vi "Write configuration.vi"(8 "error in (no error)":errorcluster, 10 "configuration":refnum<class "CEF_serializable configuration.lvclass">, 11 "DIO Instrument":refnum<class "Digital IO Instrument.lvclass">) -> (0 "error out":errorcluster, 3 "DIO Instrument out":refnum<class "Digital IO Instrument.lvclass">)   [LabVIEW 2025, in "Digital IO.lvlib" / "Digital IO Instrument.lvclass"]
uses:
  Digital IO Instrument.lvclass
  Users/Public/Documents/Sandia National Labs/TSS Plugin/CEF.lvlibp/serializable configuration/CEF_serializable configuration.lvclass
  Users/Public/Documents/Sandia National Labs/TSS Plugin/Abstract Engine.lvlibp/Plugin/Abstract/Instrument configuration/Instrument configuration.lvclass
  Digital IO Instrument.lvclass/Digital IO Instrument.ctl
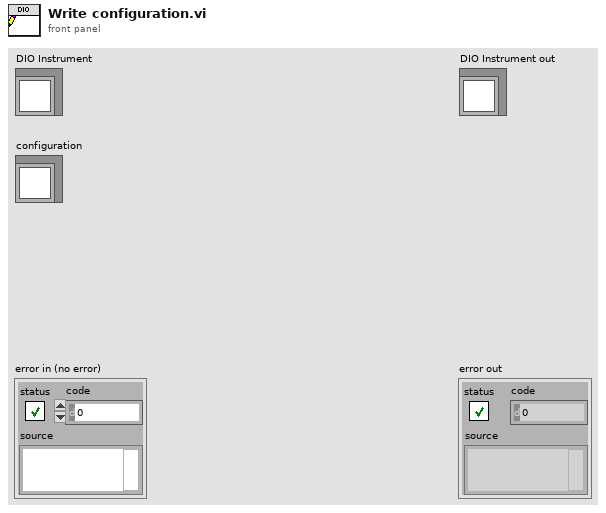
[diagram p1: front panel]
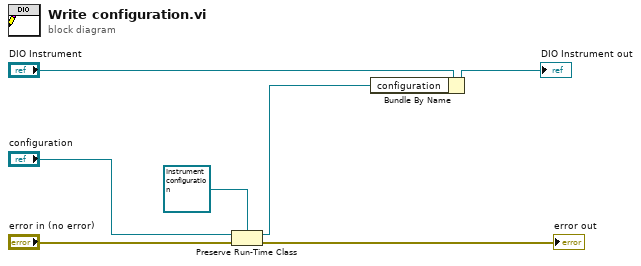
[diagram p0: block diagram]
diagram:
  n1 = Preserve Run-Time Class(object in="configuration", error in="error in (no error)", 2:refnum<class "Instrument configuration.lvclass"> refnum ("Abstract PlugIn.lvlibp:Instrument config")) -> (object out=w2:refnum<class "Instrument configuration.lvclass">, error out=→"error out":errorcluster)
  n2 = Bundle By Name(cluster="DIO Instrument", "configuration"=w2) -> (→"DIO Instrument out":refnum<class "Digital IO Instrument.lvclass">)
